vi "DAQNavi Read (Digital Wfm 1Chan 1Samp).vi"(8 "error in (no error)":errorcluster, 10 "timeout":dbl=10.0, 11 "task in":i32) -> (0 "error out":errorcluster, 2 "data":digitalwaveform(waveform)={"t0"=timestamp(0 s since 1904-01-01), "dt"=1.0, "Y"={"transitions"=[], "data"=[]}}, 3 "task out":i32)   [LabVIEW 2020]
uses:
  DAQNavi_LV.dll
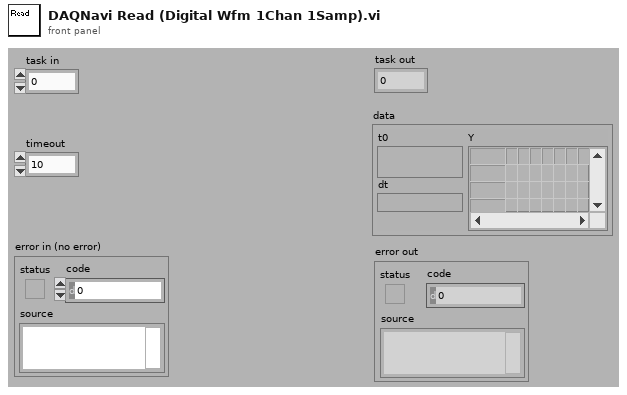
[diagram p1: front panel]
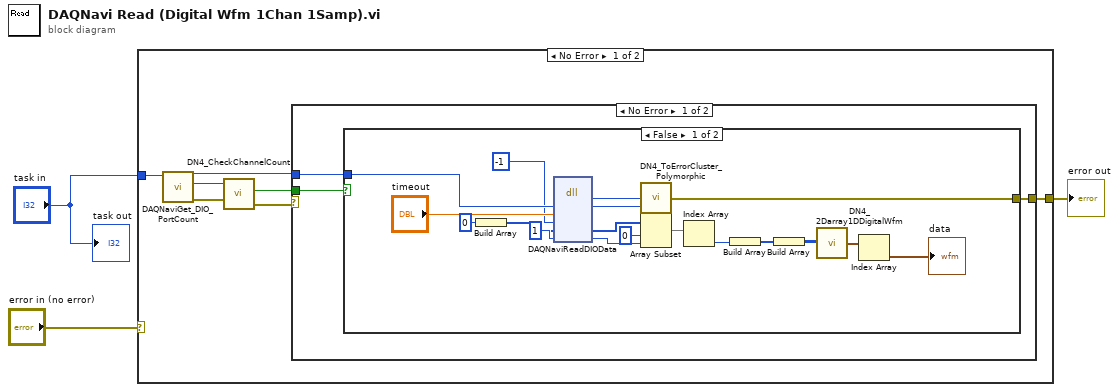
[diagram p0: block diagram]
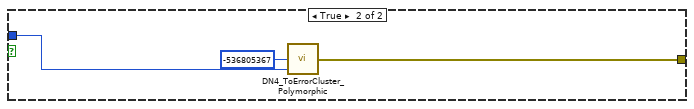
[diagram p2: hidden frame]
diagram:
  n1 = case shown="No Error" "error in (no error)" {
    selector: "error in (no error)" -> [_ w36]
    tunnel: "task in" -> [w10 _]
    tunnel: [w4 w36] -> w1
    frame No Error {
      n2 = call "DAQNaviGet_DIO_PortCount.vi"("task in"=w10) -> ("error out"=w9:errorcluster, "port count"=w8:i32, "task out"=w5:i32)  [unwired: 1 in, 7 out]
      n3 = call "DN4_CheckChannelCount.vi"("error out"=w9, "channel count"=w8) -> ("error IO"=w7:errorcluster, "greater than 1?"=w6:bool)  [unwired: 2 out]
      n4 = case shown="No Error" w7 {
        selector: w7 -> [_ w35]
        tunnel: [w13 w35] -> w4
        tunnel: w6 -> [w12 _]
        tunnel: w5 -> [w11 _]
        frame No Error {
          n5 = case shown="False" w12 {
            tunnel: [w29 w33] -> w13
            tunnel: w11 -> [w28 w32]
            frame False {
              n6 = Build Array(u8 0 ("element")) -> (w25:u8[])
              n7 = dll-call lib="DAQNavi_LV.dll" fn="DAQNaviReadDIOData"("taskID"=w28, "timeout"="timeout", "portBit"=-1, "portData"=w25, "samples"=u32 1) -> ("return type"=w30:i32, "taskID"=w15:i32, "portData"=w24:u8[], "samples"=w22:u32)  [unwired: 5 in, 2 out]
              n8 = call "DN4_ToErrorCluster_Polymorphic.vi"("task id"=w15, "error code"=w30) -> ("error out"=w29:errorcluster)  [unwired: 3 out]
              n9 = Array Subset(array=w24, index=0, length=w22) -> (w21:u8[])
              n10 = Index Array(array=w21) -> (element=w20:u8)  [unwired: 1 in]
              n11 = Build Array(w20) -> (w19:u8[])
              n12 = Build Array(w19) -> (w18:u8[][])
              n13 = call "DN4_2Darray1DDigitalWfm.vi"("data"=w18) -> ("1D Wfm"=w17:digitalwaveform[])
              n14 = Index Array(array=w17) -> (element=→"data":digitalwaveform)  [unwired: 1 in]
            }
            frame True {
              n15 = call "DN4_ToErrorCluster_Polymorphic.vi"("task id"=w32, "error code"=-536805367 ("error code (0)")) -> ("error out"=w33:errorcluster)  [unwired: 3 out]
            }
          }
        }
        frame Error {
        }
      }
    }
    frame Error {
    }
  }
  "error out" <- w1
  "task out" <- "task in"
